vi "Set Controls RegisterMap.vi"(8 "error in (no error)":errorcluster, 10 "Controls RegisterMap":T2[](array[typedef]) {"Address" format="%.0x"}, 11 "Item Ref in":T1 format="%.0x") -> (0 "error out":errorcluster, 3 "Item Ref out":T1 format="%.0x")   [LabVIEW 2016, in "FPGA Addon System Explorer.lvlib"]
uses:
  <vilib>/rvi/Bitfile/nirviControlStructure.ctl
  <vilib>/rvi/Bitfile/nirviTypdefDescription.ctl
  <vilib>/rvi/Bitfile/nirviMechanicalAction.ctl
  <vilib>/rvi/Bitfile/nirviSubControlStructure.ctl
  <vilib>/rvi/Bitfile/nirviClusterElementControl.ctl
  <vilib>/NI Veristand/Custom Device API/Custom Device Item Ref.ctl
  <vilib>/NI Veristand/Custom Device API/Set Item Property (Variant).vi
  Shared/Constants.vi
  FPGA Addon System Explorer.lvlib
  <vilib>/NI VeriStand/Custom Device API/Custom Device API.lvlib
  Shared/FPGA Addon Shared.lvlib
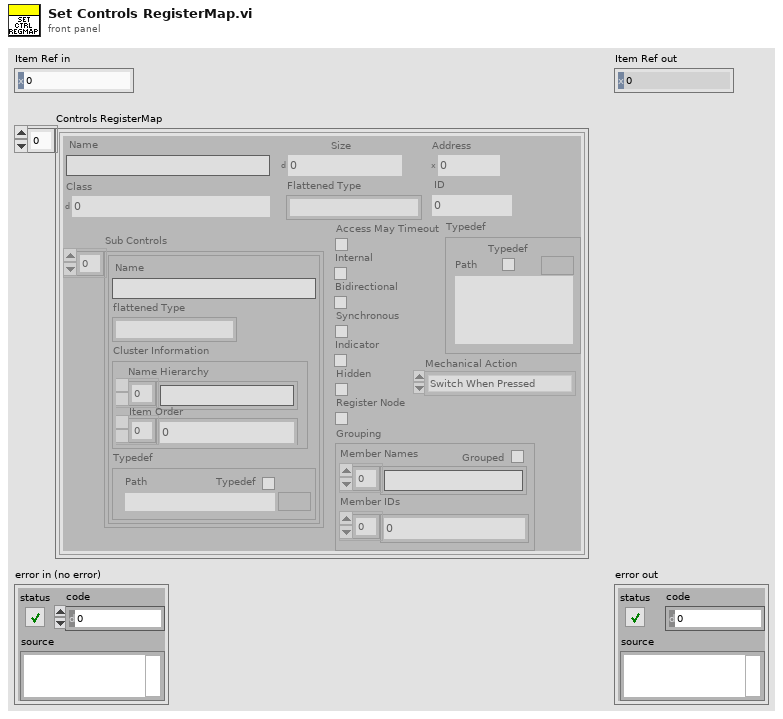
[diagram p1: front panel]
types:
  T1 = typedef "Custom Device API.lvlib/Custom Device Item Ref.ctl" = u64
  T2 = typedef "nirviControlStructure.ctl" = cluster{"Name":string, "Hidden":bool, "Indicator":bool, "Flattened Type":string, "Grouping":cluster{"Grouped":bool, "Member Names":string[], "Member IDs":u32[]}, "Address":u32, "Size":u32, "Class":u32, "Internal":bool, "Typedef":T3, "ID":u32, "Bidirectional":bool, "Synchronous":bool, "Mechanical Action":T4, "Sub Controls":T5[], "Access May Timeout":bool, "Register Node":bool}
  T3 = typedef "nirviTypdefDescription.ctl" = cluster{"Typedef":bool, "Path":path}
  T4 = typedef "nirviMechanicalAction.ctl" = enum8{"Switch When Pressed", "Switch When Released", "Switch Until Released", "Latch When Pressed", "Latch When Released", "Latch Until Released"}
  T5 = typedef "nirviSubControlStructure.ctl" = cluster{"Name":string, "flattened Type":string, "Cluster Information":T6, "Typedef":T3}
  T6 = typedef "nirviClusterElementControl.ctl" = cluster{"Name Hierarchy":string[], "Item Order":u32[]}
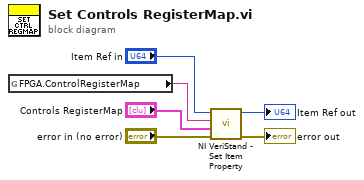
[diagram p0: block diagram]
diagram:
  n1 = global read "Constants.vi" "FPGA.ControlRegisterMap"() -> (w3:string)
  n2 = call-poly <vilib>:"NI VeriStand - Set Item Property.vi"("error in (no error)"="error in (no error)", "Value"="Controls RegisterMap", "Property Name"=w3, "Item Ref in"="Item Ref in") -> ("error out"=→"error out":errorcluster, "Item Ref out"=→"Item Ref out":T1)  [unwired: 5 in, 1 out]
